vi "CCD Acquire Image.vi"(8 "error in":errorcluster) -> (0 "error out":errorcluster, 3 "Intensity Graph":dbl[][](graph))   [LabVIEW 2020, in "Examples.lvlib"]
doc: "Example for a CCD spectrum acquisition."
uses:
  Examples.lvlib
  Classes/CCD/CCD.lvclass
  4aef6941-9f58-45d1-a797-2b486d7897ac.vi
  <vilib>/Utility/file.llb/Write Delimited Spreadsheet (DBL).vi
panel:
  # "Connector Pane"
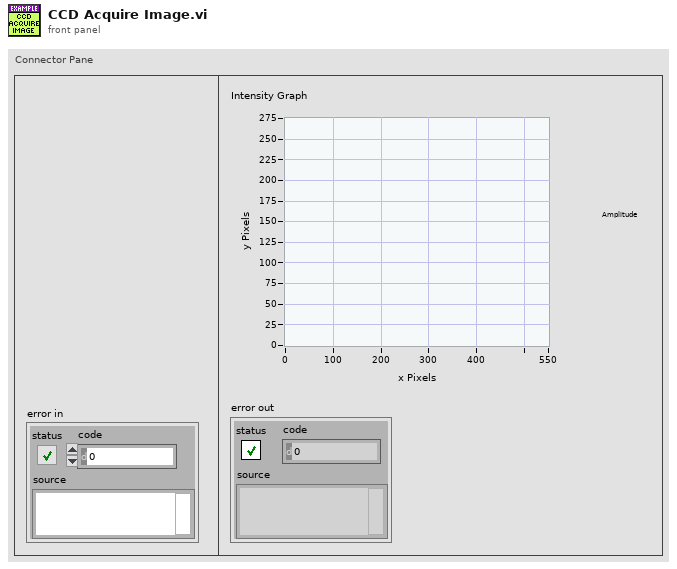
[diagram p1: front panel]
types:
  T1 = cluster{"ROI-index":i32, "xOrigin":i32, "yOrigin":i32, "xSize":i32, "ySize":i32, "xBin":i32, "yBin":i32}
  T2 = typedef "horiba.lvlib/CCD.lvclass/ccdAcquisitionData.ctl" = cluster{"acqIndex":i32, "ROIs":T3[], "timestamp":string}
  T3 = typedef "horiba.lvlib/CCD.lvclass/imageAcqData.ctl" = cluster{"roiMetaData":T4, "xAxis":dbl[], "yData":dbl[][]}
  T4 = typedef "horiba.lvlib/CCD.lvclass/roiMetaData.ctl" = cluster{"roiIndex":i32, "xBinning":i32, "xOrigin":i32, "xSize":i32, "yBinning":i32, "yOrigin":i32, "ySize":i32}
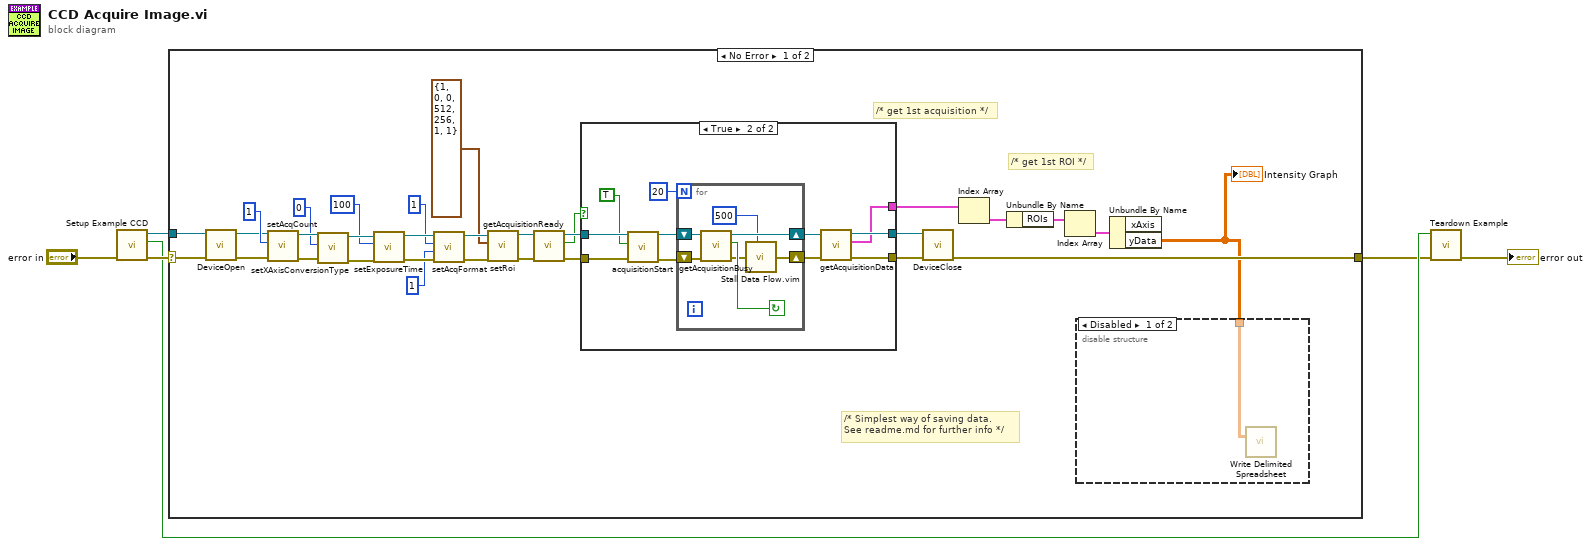
[diagram p0: block diagram]
diagram:
  n1 = call "Setup Example CCD.vi"("error in (no error)"="error in") -> ("error out"=w4:errorcluster, "Module Was Already Running?"=w2:bool, "CCD out"=w3:refnum<class "CCD.lvclass">)  [unwired: 8 in]
  n2 = case shown="No Error" w4 {
    selector: w4 -> [w37 w59]
    tunnel: w3 -> [w8 _]
    tunnel: [w16 w59] -> w1
    frame No Error {
      # "/* Simplest way of saving data.\nSee readme.md for further info */"
      # "/* get 1st ROI */"
      # "/* get 1st acquisition */"
      n3 = call-dynamic "DeviceOpen.vi"("error in (no error)"=w37, "CCD in"=w8) -> ("error out"=w9:errorcluster, "CCD out"=w7:refnum<class "CCD.lvclass">)  [unwired: 6 in, 2 out]
      n4 = call "setAcqCount.vi"("error in (no error)"=w9, "count"=1, "CCD in"=w7) -> ("error out"=w35:errorcluster, "CCD out"=w34:refnum<class "CCD.lvclass">)  [unwired: 5 in, 2 out]
      n5 = call "setXAxisConversionType.vi"("error in (no error)"=w35, "type"=0, "CCD in"=w34) -> ("error out"=w32:errorcluster, "CCD out"=w31:refnum<class "CCD.lvclass">)  [unwired: 5 in, 2 out]
      n6 = call "setExposureTime.vi"("error in (no error)"=w32, "exposure time [ms] or [us]"=100, "CCD in"=w31) -> ("error out"=w29:errorcluster, "CCD out"=w28:refnum<class "CCD.lvclass">)  [unwired: 5 in, 2 out]
      n7 = call "setAcqFormat.vi"("error in (no error)"=w29, "format"=1, "number of ROIs"=1, "CCD in"=w28) -> ("error out"=w25:errorcluster, "CCD out"=w24:refnum<class "CCD.lvclass">)  [unwired: 4 in, 2 out]
      n8 = call "setRoi.vi"("error in (no error)"=w25, "roiConfig"=T1 {"ROI-index"=1, "xOrigin"=0, "yOrigin"=0, "xSize"=512, "ySize"=256, "xBin"=1, "yBin"=1}, "CCD in"=w24) -> ("error out"=w22:errorcluster, "CCD out"=w21:refnum<class "CCD.lvclass">)  [unwired: 5 in, 2 out]
      n9 = call "getAcquisitionReady.vi"("error in (no error)"=w22, "CCD in"=w21) -> ("error out"=w20:errorcluster, "ready"=w18:bool, "CCD out"=w19:refnum<class "CCD.lvclass">)  [unwired: 7 in]
      n10 = case shown="True" w18 {
        tunnel: w20 -> [w39 w51]
        tunnel: w19 -> [w40 w50]
        tunnel: [w39 w44] -> w17
        tunnel: [w40 w42] -> w15
        tunnel: [_ w41] -> w12
        frame False {
        }
        frame True {
          n11 = call "acquisitionStart.vi"("error in (no error)"=w51, "openShutter"=TRUE, "CCD in"=w50) -> ("error out"=w46:errorcluster, "CCD out"=w45:refnum<class "CCD.lvclass">)  [unwired: 5 in, 2 out]
          n12 = for {
            N: 20 -> [_]
            shift-right: [w54] -> w47
            shift-left: w46 -> [w57]
            shift-right: [w53] -> w43
            shift-left: w45 -> [w58]
            stop <- w56 continue-if-true
            n13 = call "getAcquisitionBusy.vi"("error in (no error)"=w57, "CCD in"=w58) -> ("error out"=w55:errorcluster, "isBusy"=w56:bool, "CCD out"=w53:refnum<class "CCD.lvclass">)  [unwired: 7 in]
            n14 = call "Stall Data Flow.vim"("value in"=w55, "milliseconds to wait"=u32 500) -> ("value out"=w54:errorcluster)  [unwired: 1 out]
          }
          n15 = call "getAcquisitionData.vi"("error in (no error)"=w47, "CCD in"=w43) -> ("error out"=w44:errorcluster, "ccdAcquisitions"=w41:T2[], "CCD out"=w42:refnum<class "CCD.lvclass">)  [unwired: 6 in, 1 out]
        }
      }
      n16 = call-dynamic "DeviceClose.vi"("error in (no error)"=w17, "CCD in"=w15) -> ("error out"=w16:errorcluster)  [unwired: 5 in, 4 out]
      n17 = Index Array(array=w12) -> (element=w11:T2)  [unwired: 1 in]
      n18 = Unbundle By Name(w11) -> ("ROIs"=w14:T3[])
      n19 = Index Array(array=w14) -> (element=w13:T3)  [unwired: 1 in]
      n20 = Unbundle By Name(w13) -> ("yData"=w10:dbl[][])  [unwired: 1 out]
      "Intensity Graph" <- w10
      n21 = disable-structure shown="Disabled" {
        disable-tunnel: w10 -> [w38 _]
        frame Disabled {
          n22 = call-poly <vilib>:"Write Delimited Spreadsheet.vi"("2D data"=w38) -> ()  [unwired: 13 in, 2 out]
        }
        frame Enabled {
        }
      }
    }
    frame Error {
    }
  }
  n23 = call "Teardown Example.vi"("error in (no error)"=w1, "Module Was Already Running?"=w2) -> ("error out"=→"error out":errorcluster)  [unwired: 9 in]
